vi "RT-Init.vi"() -> (0 "Weights":T1, 1 "Data-in Settings":T3, 2 "Motor-Controller Settings":T2)   [LabVIEW 2020]
uses:
  <vilib>/FPGAPlugInAG/roboRIO/niLvFpga_Open_roboRIO.vi
  <vilib>/rvi/interface/common/dynamic/niFpgaDynamicAddResources.vi
  <vilib>/rvi/interface/nirviOpenFPGA/nirviOpenFPGA.xnode
  FPGA Bitfiles/exo1_FPGATarget_DataIn_R1wp+qdUXdo.lvbitx
  DataIn.vi
panel:
  in  "Weights (4x9)":dbl[][](array[numeric])
  in  "Weights (1000x2001)":dbl[][](array[numeric])
  in  "Weights (4x4x8)":dbl[][][](array[numeric])
  in  "Weights (4x4x15)":dbl[][][](array[numeric])
  in  "Hexadecimal?":bool
  in  "Number of Frames to Display":i32=15
  in  "receive queue size":u32=5
  in  "baud rate":u32=125000
  in  "interface index":u32
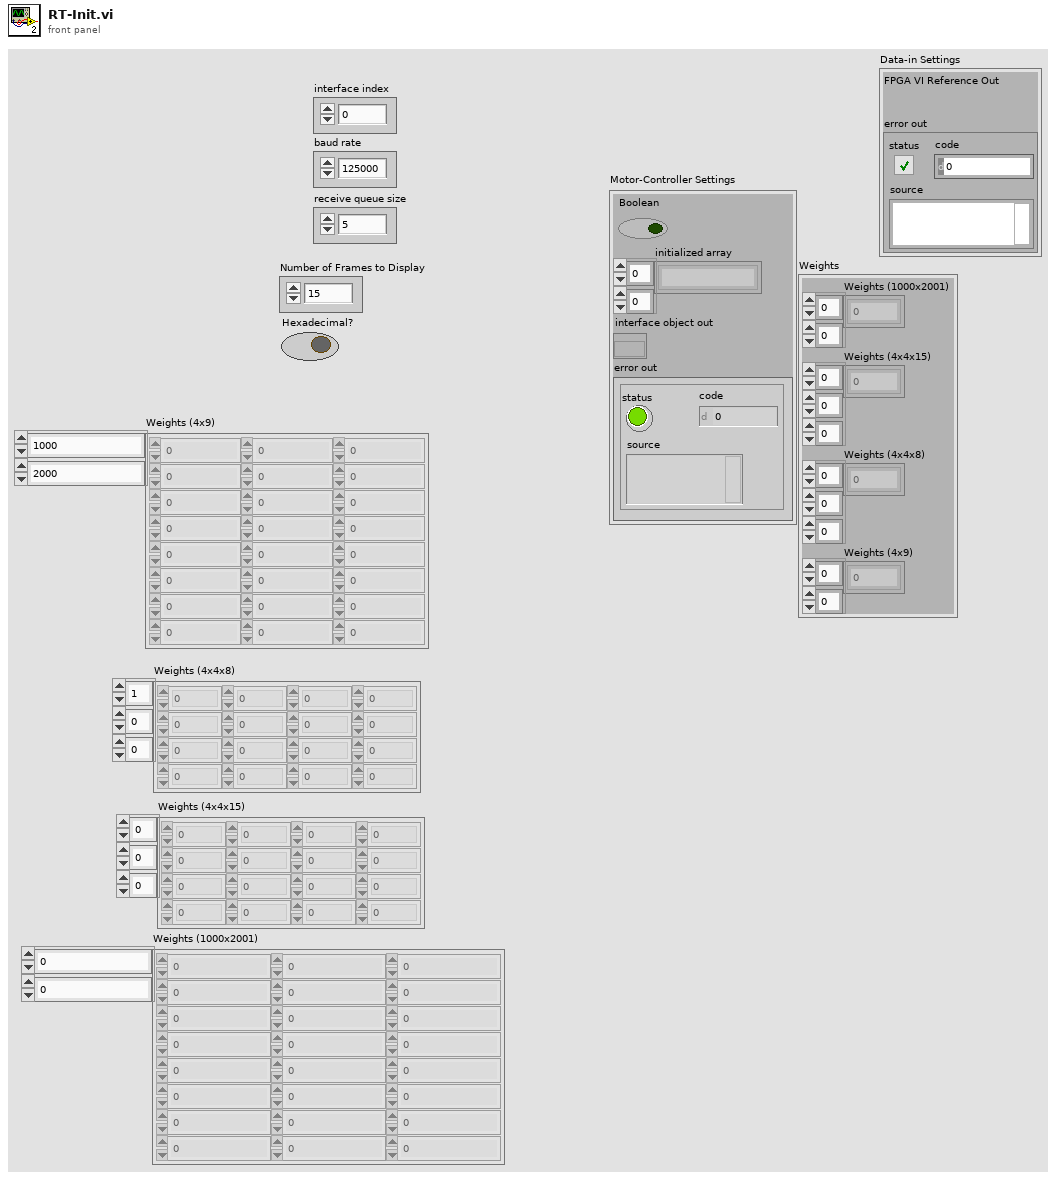
[diagram p1: front panel]
types:
  T1 = cluster{"Weights (1000x2001)":dbl[][], "Weights (4x4x15)":dbl[][][], "Weights (4x4x8)":dbl[][][], "Weights (4x9)":dbl[][]}
  T2 = cluster{"Boolean":bool, "initialized array":string[][], "interface object out":refnum<k20>, "error out":errorcluster}
  T3 = cluster{"FPGA VI Reference Out":refnum<k20>, "error out":errorcluster}
  T4 = cluster{"Hexadecimal?":bool, string[][], "interface object out":refnum<k20>, "error out":errorcluster}
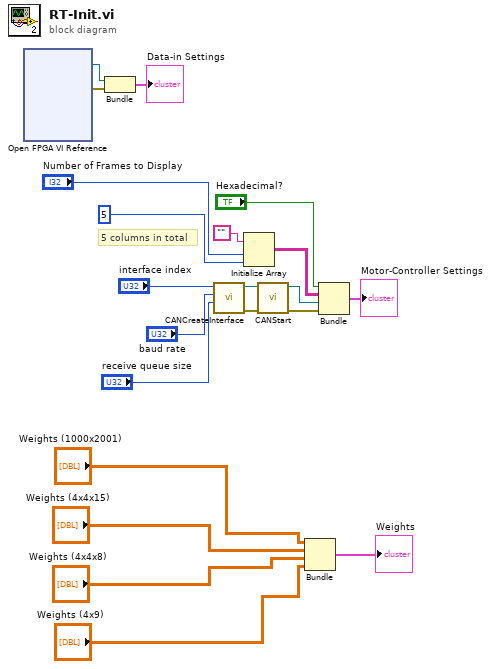
[diagram p0: block diagram]
diagram:
  # "5 columns in total"
  n1 = xnode "Open FPGA VI Reference"() -> ("FPGA VI Reference Out"=w9:refnum<k20>, "error out"=w8:errorcluster)  [unwired: 2 in]
  n2 = Bundle("FPGA VI Reference Out"=w9, "error out"=w8) -> (→"Data-in Settings":T3)  [unwired: 1 in]
  n3 = call <vilib>:"CANCreateInterface.vi"("receive queue size (5)"="receive queue size", "baud rate (125000 bps)"="baud rate", "interface index"="interface index") -> ("error out"=w21:errorcluster, "interface object out"=w20:refnum<k20>)  [unwired: 7 in]
  n4 = Initialize Array("" ("Empty String Constant"), "Number of Frames to Display", 5 ("dimension size")) -> (w12:string[][])
  n5 = call <vilib>:"CANStart.vi"("error in (no error)"=w21, "interface object in"=w20) -> ("error out"=w10:errorcluster, "interface object out"=w11:refnum<k20>)  [unwired: 8 in]
  n6 = Bundle("Weights (1000x2001)"="Weights (1000x2001)", "Weights (4x4x15)"="Weights (4x4x15)", "Weights (4x4x8)"="Weights (4x4x8)", "Weights (4x9)"="Weights (4x9)") -> (→"Weights":T1)  [unwired: 1 in]
  n7 = Bundle("Hexadecimal?"="Hexadecimal?", w12, "interface object out"=w11, "error out"=w10) -> (→"Motor-Controller Settings":T4)  [unwired: 1 in]
